vi "Initialize.vi"(8 "error in (no error)":errorcluster, 10 "DeviceName":string, 11 "PointGrey in":refnum<class "MoveDataFile.lvclass">) -> (0 "error out":errorcluster, 1 "new command(s)":string, 2 "DeviceName":string, 3 "PointGrey out":refnum<class "MoveDataFile.lvclass">)   [LabVIEW 2011, in "MoveDataFile.lvclass"]
uses:
  MoveDataFile.lvclass
  BaseDriver/BaseDriver.lvclass
  MoveDataFile.lvclass/MoveDataFile.ctl
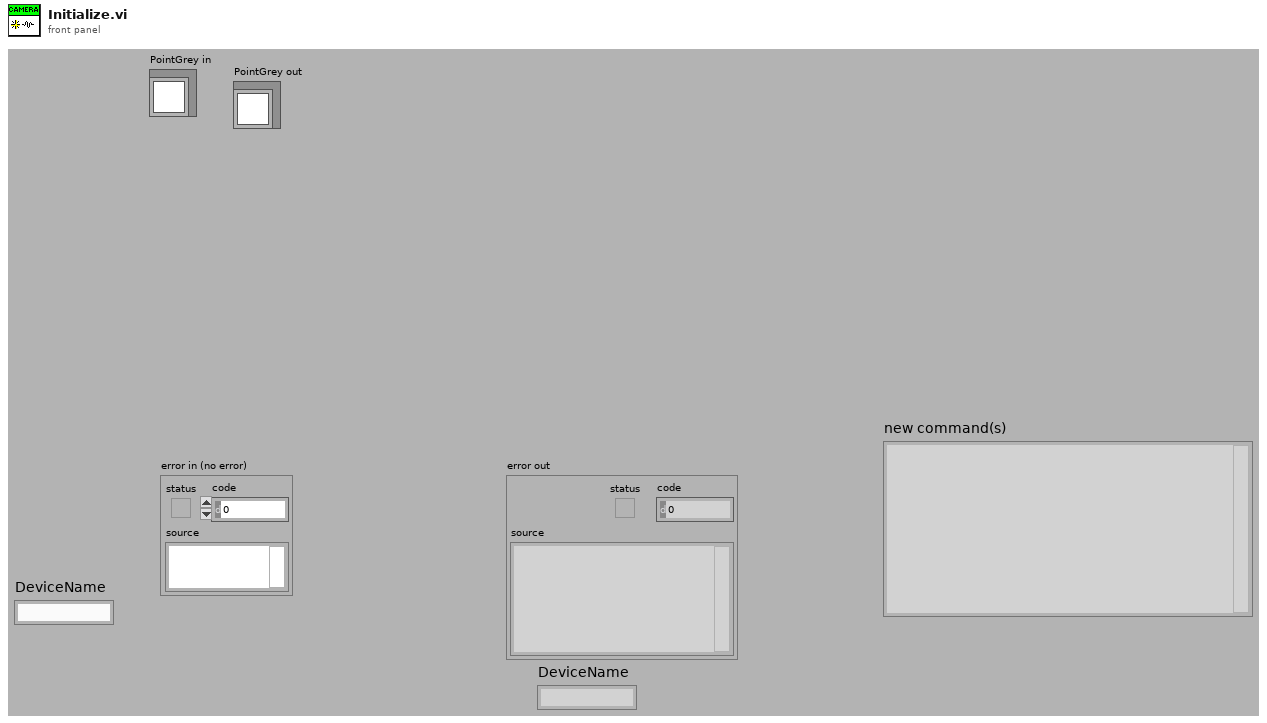
[diagram p1: front panel]
types:
  T1 = typedef "MoveDataFile.lvclass/SettingsTypdef.ctl" = cluster{"FileExtension":string, "FileSourcePath":path, "DeleteSource":T2, "Save":T2, "LocalSavingPath":path, "maxshot#":dbl}
  T2 = typedef "OnOffTypeDef.ctl" = enum16{"off", "on"}
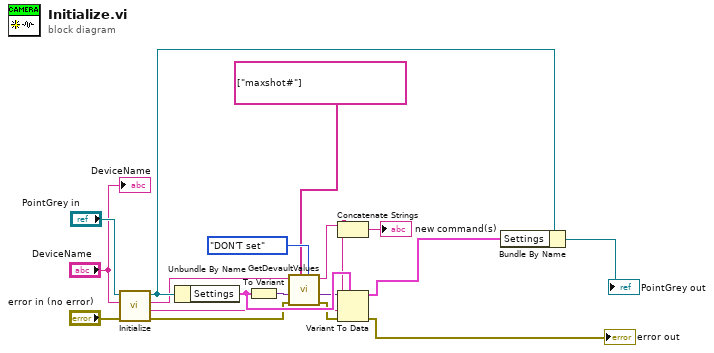
[diagram p0: block diagram]
diagram:
  n1 = call-parent "Initialize.vi"("error in (no error)"="error in (no error)", "DeviceName"="DeviceName", "BaseDriver in"="PointGrey in") -> ("error out"=w6:errorcluster, "new command(s)"=w7:string, "DeviceName"=w8:string, "BaseDriver out"=w11:refnum<class "MoveDataFile.lvclass">)  [unwired: 5 in]
  n2 = Unbundle By Name(w11) -> ("Settings"=w15:T1)
  n3 = To Variant(anything=w15) -> (Variant=w16:variant)
  n4 = call "GetDevaultValues.vi"("set or DON'T set"=enum16{"set", "DON'T set"}."DON'T set", "set following Variables (empty = all avriables)"=string[] ["maxshot#"], "error in (no error)"=w6, "variant"=w16, "Device Name"=w8) -> ("error out"=w5:errorcluster, "variant out"=w14:variant, "new command(s)"=w12:string)  [unwired: 4 in]
  n5 = Concatenate Strings(w12, w7) -> (→"new command(s)":string)
  n6 = Variant To Data(error in=w5, type=w15, Variant=w14) -> (data=w13:T1, error out=→"error out":errorcluster)
  n7 = Bundle By Name(cluster=w11, "Settings"=w13) -> (→"PointGrey out":refnum<class "MoveDataFile.lvclass">)
  "DeviceName" <- "DeviceName"
